vi "SHOW SPECIAL.vi"(8 "error in (no error)":errorcluster, 11 "VISA resource name":refnum<visa-resource-name>) -> (0 "error out":errorcluster, 1 "Serial Number":string, 2 "read buffer":string, 3 "VISA resource name out":refnum<visa-resource-name>)   [LabVIEW 2019, in "AH2500.lvlib"]
uses:
  AH2500.lvlib
panel:
  # "SHOW SPECIAL"
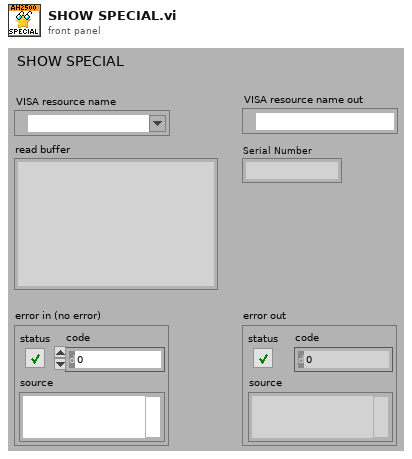
[diagram p1: front panel]
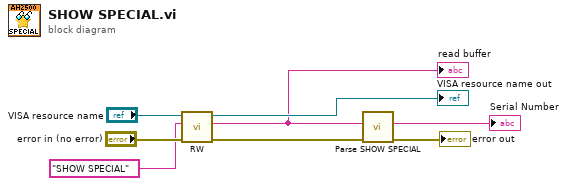
[diagram p0: block diagram]
diagram:
  n1 = call "RW.vi"("error in (no error)"="error in (no error)", "write buffer"="SHOW SPECIAL", "VISA Refnum in"="VISA resource name") -> ("error out"=w3:errorcluster, "read buffer"=w2:string, "VISA Refnum out"=→"VISA resource name out":refnum<visa-resource-name>)  [unwired: 6 in]
  "read buffer" <- w2
  n2 = call "Parse SHOW SPECIAL.vi"("error in"=w3, "read buffer"=w2) -> ("error out"=→"error out":errorcluster, "Serial Number"=→"Serial Number":string)  [unwired: 8 in]
